vi "General Error Handler.vi"(0 "[error code] (0)":i32 format="%0.0f", 1 "[user-defined codes]":i32[](array[numeric]), 2 "[user-defined descriptions]":string[](array[string]), 5 "[error source] (\" \")":string, 9 "type of dialog (OK msg:1)":T1=1 items=["no dialog", "OK message", "continue or stop message", "OK message + warnings", "continue/stop + warnings"], 11 "error in (no error)":errorcluster, 12 "[exception action] (none:0)":i32(ring) items=["no exception", "cancel error on match", "set error on match"], 13 "[exception code]":i32 format="%0.0f", 14 "[exception source]":string) -> (4 "error?":bool, 6 "code out":i32 format="%0.0f", 8 "source out":string, 10 "message":string=" INSTRUCTIONS:\r\rNormal Use:  When using subVIs that incorporate the error in/error out (or error I/O) structure, place this handler where you want to inform the user of an error, typically at the end of the I/O data path, as the last action of the program.  If the error in error? is ERROR, the handler creates a message describing the error and its source.  If the type of dialog = 1 (default), the message is displayed to the user, who can only acknowedge it.  If the type = 2, the user can acknowledge the message or abort execution; aborting a program with active I/O is not recommended.  If the type = 0, no message is displayed; this is used to process the error programmatically, and the error out cluster elements are wired to individual terminals for that reason.  \r\rOther Use:\n\r\nlocal testing.  To test the error code of a subVI or function that does not have the error I/O structure, you can wire its error code and a source string to the local error code and error source inputs.  If error in error? indicates no error and error code is not equal to 0, the local code and source are substituted for the error in values, and error? is set TRUE (ERROR).", 15 "error out":errorcluster)   [LabVIEW 2013]
doc: "Indicates whether an error occurred. If an error occurred, this VI returns a description of the error and optionally displays a dialog box."
uses:
  DialogType.ctl
  DialogTypeEnum.ctl
panel:
  # "Reinitialize to default to display instructions."
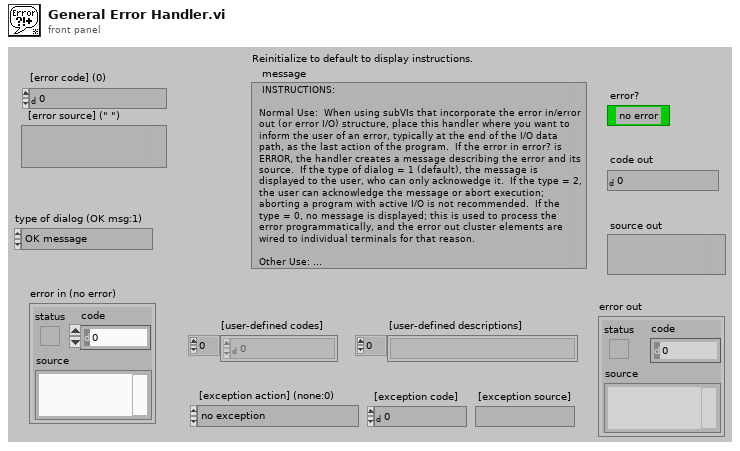
[diagram p1: front panel]
types:
  T1 = typedef "DialogType.ctl" = u16
  T2 = typedef "DialogTypeEnum.ctl" = enum16{"no dialog", "OK message", "continue or stop message", "auto error handling dialog", "OK message + warnings", "continue/stop + warnings"}
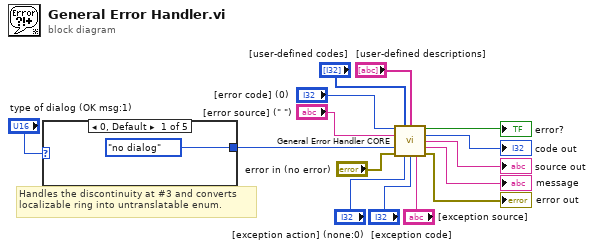
[diagram p0: block diagram]
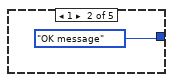
[diagram p2: hidden frame]
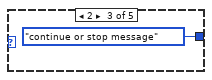
[diagram p3: hidden frame]
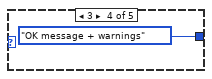
[diagram p4: hidden frame]
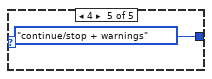
[diagram p5: hidden frame]
diagram:
  # "Handles the discontinuity at #3 and converts\nlocalizable ring into untranslatable enum."
  n1 = case shown="0, Default" "type of dialog (OK msg:1)" {
    tunnel: [DialogTypeEnum."no dialog" ("type of dialog (OK msg:1)") DialogTypeEnum."OK message" ("type of dialog (OK msg:1)") DialogTypeEnum."continue or stop message" ("type of dialog (OK msg:1)") DialogTypeEnum."OK message + warnings" ("type of dialog (OK msg:1)") DialogTypeEnum."continue/stop + warnings" ("type of dialog (OK msg:1)")] -> w1
    frame 0, Default {
    }
    frame 1 {
    }
    frame 2 {
    }
    frame 3 {
    }
    frame 4 {
    }
  }
  n2 = call "General Error Handler CORE.vi"("[error code] (0)"="[error code] (0)", "[user-defined codes]"="[user-defined codes]", "[user-defined descriptions]"="[user-defined descriptions]", "[error source] (\" \")"="[error source] (\" \")", "type of dialog (OK msg:1)"=w1, "error in (no error)"="error in (no error)", "[exception action] (none:0)"="[exception action] (none:0)", "[exception code]"="[exception code]", "[exception source]"="[exception source]") -> ("error?"=→"error?":bool, "code out"=→"code out":i32, "source out"=→"source out":string, "message"=→"message":string, "error out"=→"error out":errorcluster)  [unwired: 1 in, 1 out]
